vi "Error Correction (SubVI).vi"(11 "Cluster":T2) -> (3 "cluster":T1)   [LabVIEW 2014]
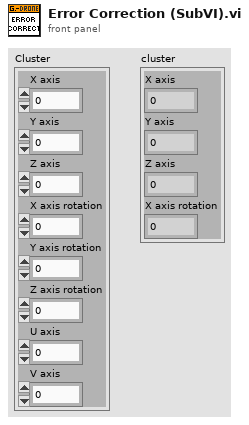
[diagram p1: front panel]
types:
  T1 = cluster{"X axis":dbl, "Y axis":dbl, "Z axis":dbl, "X axis rotation":dbl}
  T2 = cluster{"X axis":dbl, "Y axis":dbl, "Z axis":dbl, "X axis rotation":dbl, "Y axis rotation":dbl, "Z axis rotation":dbl, "U axis":dbl, "V axis":dbl}
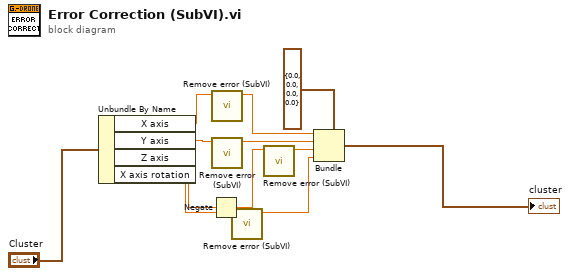
[diagram p0: block diagram]
diagram:
  n1 = Unbundle By Name("Cluster") -> ("X axis"=w5:dbl, "Y axis"=w7:dbl, "Z axis"=w4:dbl, "X axis rotation"=w9:dbl)
  n2 = Negate(x=w4) -> (-x=w8:dbl)
  n3 = call "Remove error (SubVI).vi"("X axis in"=w5) -> ("X axis out"=w6:dbl)  [unwired: 10 in]
  n4 = call "Remove error (SubVI).vi"("X axis in"=w7) -> ("X axis out"=w10:dbl)  [unwired: 10 in]
  n5 = call "Remove error (SubVI).vi"("X axis in"=w9) -> ("X axis out"=w12:dbl)  [unwired: 10 in]
  n6 = call "Remove error (SubVI).vi"("X axis in"=w8) -> ("X axis out"=w11:dbl)  [unwired: 10 in]
  n7 = Bundle(cluster=T1 {"X axis"=0.0, "Y axis"=0.0, "Z axis"=0.0, "X axis rotation"=0.0}, "X axis"=w6, "Y axis"=w10, "Z axis"=w11, "X axis rotation"=w12) -> (→"cluster":T1)
